vi "E1.vi"() -> ()   [LabVIEW 2018]
panel:
  out "Waveform Graph":dbl[](graph)
  in  "Knob":dbl(knob) scale=0.0..10.0
  in  "Amplitude":dbl
  in  "Sampling freq":dbl
  in  "Frequency":dbl
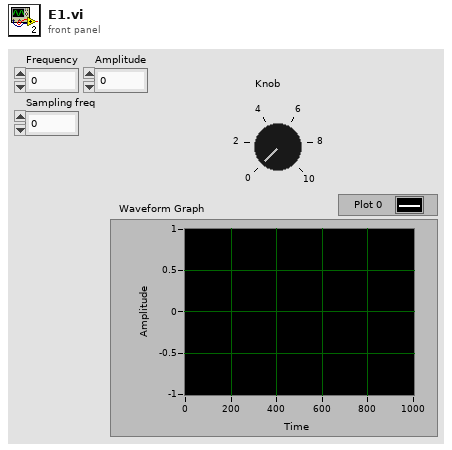
[diagram p1: front panel]
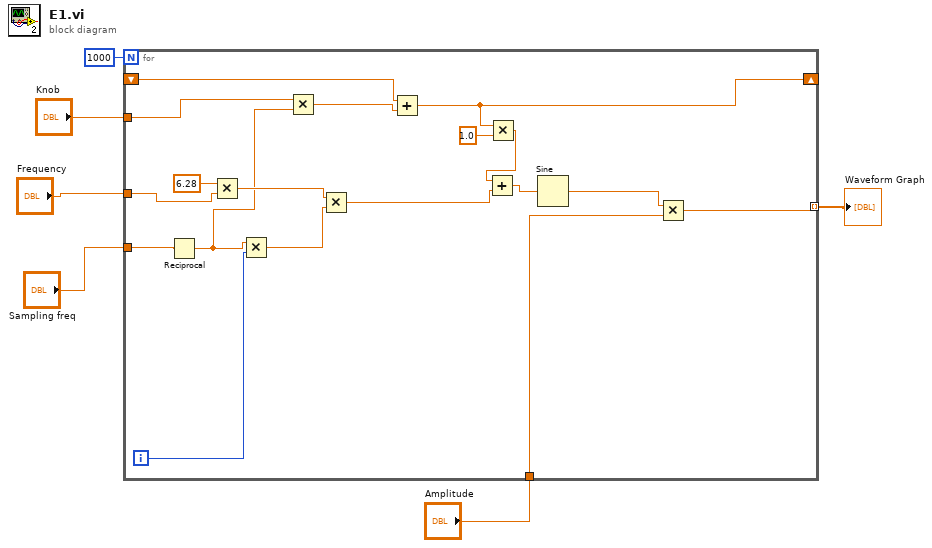
[diagram p0: block diagram]
diagram:
  n1 = for {
    N: 1000 -> [_]
    tunnel: "Frequency" -> [w21]
    tunnel: "Sampling freq" -> [w23]
    tunnel: "Amplitude" -> [w18]
    tunnel: "Knob" -> [w17]
    shift-right: [w13] -> _
    shift-left: _ -> [w14]
    tunnel: [w7] -> w2 mode=indexing
    i -> [w22]
    n2 = Reciprocal(x=w23) -> (1/x=w16:dbl)
    n3 = Multiply(x=6.28, y=w21) -> (x*y=w20:dbl)
    n4 = Multiply(x=w16, y=w22) -> (x*y=w19:dbl)
    n5 = Multiply(x=w17, y=w16) -> (x*y=w15:dbl)
    n6 = Multiply(x=w20, y=w19) -> (x*y=w8:dbl)
    n7 = Add(x=w14, y=w15) -> (x+y=w13:dbl)
    n8 = Multiply(x=w13, y=1.0) -> (x*y=w9:dbl)
    n9 = Add(x=w9, y=w8) -> (x+y=w10:dbl)
    n10 = Sine(x=w10) -> (sin(x)=w11:dbl)
    n11 = Multiply(x=w11, y=w18) -> (x*y=w7:dbl)
  }
  "Waveform Graph" <- w2
